vi "salProcessorStandby.vi"(8 "error in (no error)":errorcluster, 11 "SALCommunicatorController in":refnum<class "SALCommunicatorController.lvclass">) -> (0 "error out":errorcluster, 3 "SALCommunicatorController out":refnum<class "SALCommunicatorController.lvclass">)   [LabVIEW 2016, in "SALCommunicatorController.lvclass"]
uses:
  SALCommunicatorController.lvclass
  ts_sallv_exa/SALLV_EXA.lvlib
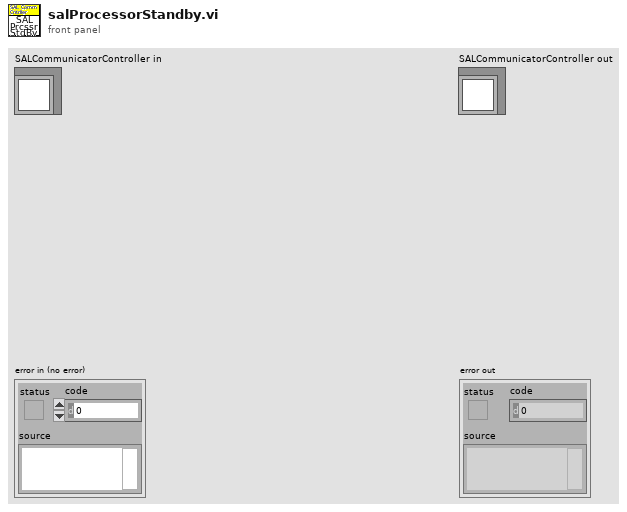
[diagram p1: front panel]
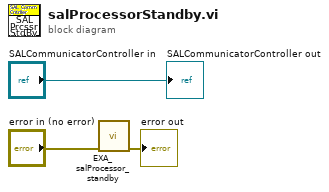
[diagram p0: block diagram]
diagram:
  n1 = call "EXA_salProcessor_standby.vi"("error in (no error)"="error in (no error)") -> ("error out"=→"error out":errorcluster)  [unwired: 9 in, 1 out]
  "SALCommunicatorController out" <- "SALCommunicatorController in"
